vi "BangBang_GetAll.vi"(11 "BANG_BANG":T1 {"Measurment" format="%13.5p"; "Setpoint" format="%13.5p"; "Tolerance" format="%13.5p"}) -> (1 "Tolerance":dbl, 2 "Measurment":dbl, 3 "Setpoint":dbl)   [LabVIEW 2019, in "Trajectory_Library.lvlib"]
doc: "Gets elements of the internal data cluster\n\nInput:\n - BangBang -- Data cluster\n\nOutput\n - Setpoint -- Current stored setpoint (SP)\n - Measurement -- Current stored process variable (PV)\n - Tolerance -- Current stored tolerance."
uses:
  Trajectory_Library.lvlib
  TypeDef/BANG_BANG.ctl
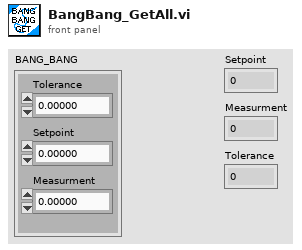
[diagram p1: front panel]
types:
  T1 = typedef "Trajectory_Library.lvlib/BANG_BANG.ctl" = cluster{"Tolerance":dbl, "Setpoint":dbl, "Measurment":dbl}
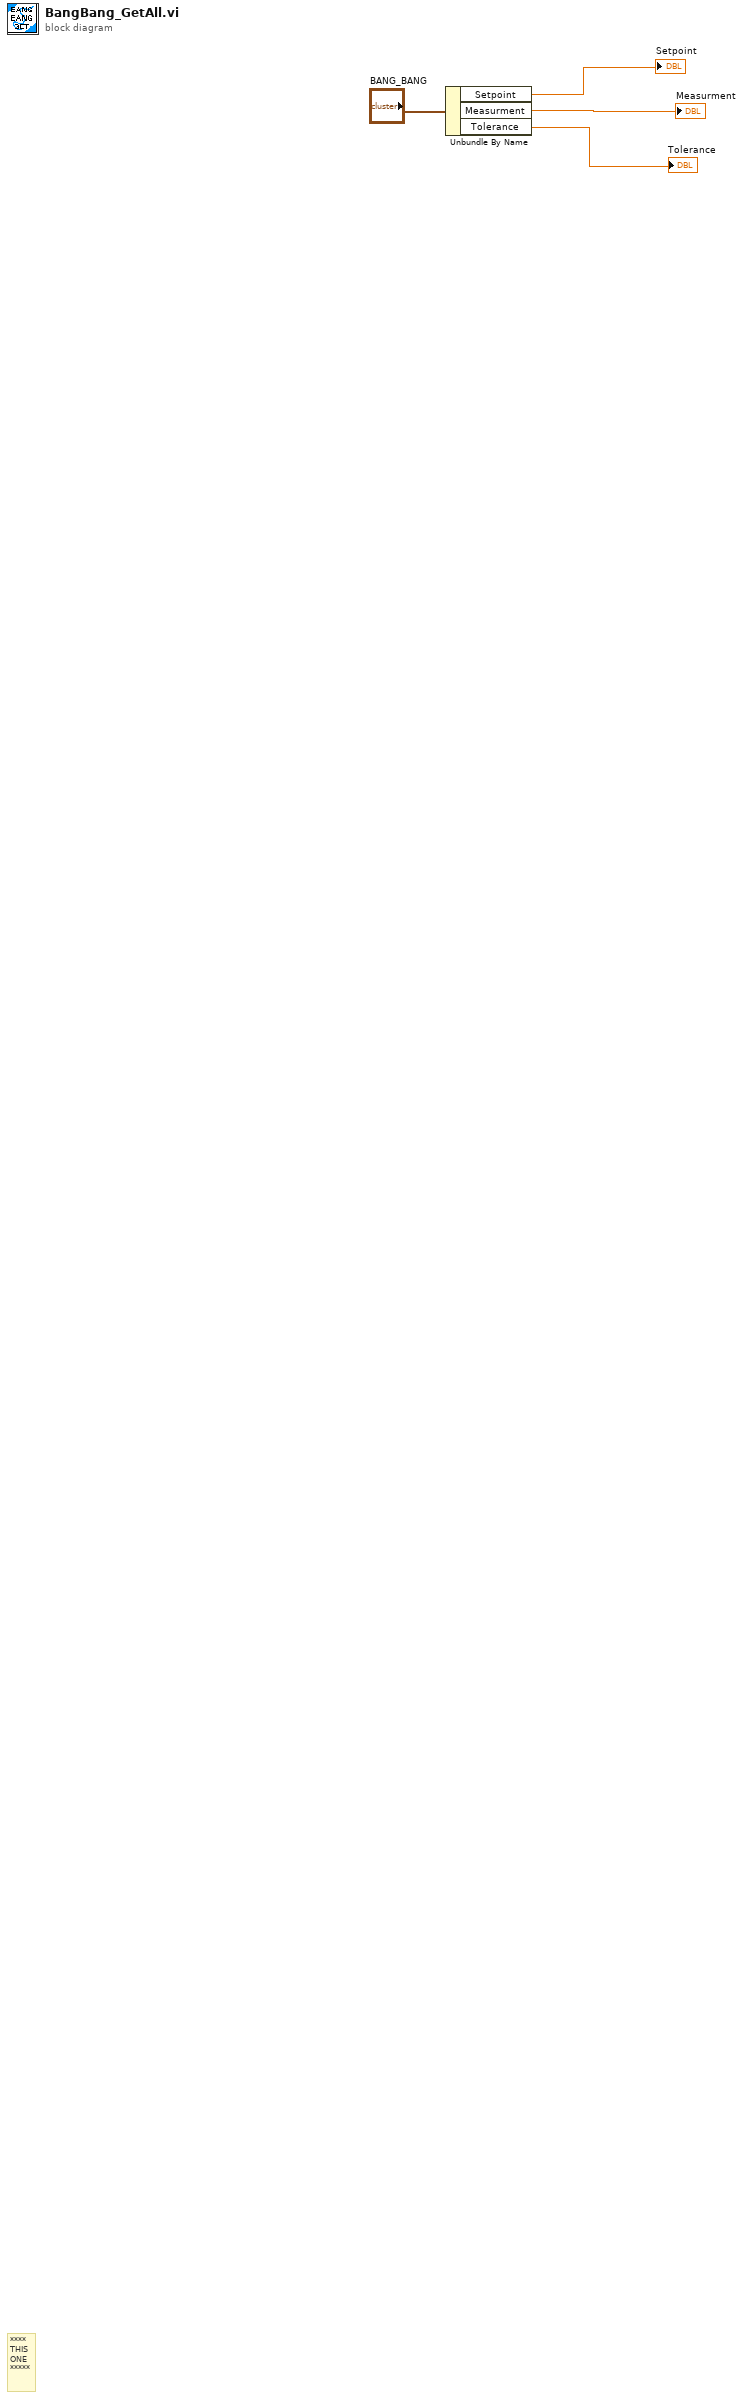
[diagram p0: block diagram]
diagram:
  # "****\nTHIS\nONE\n*****"
  n1 = Unbundle By Name("BANG_BANG") -> ("Setpoint"=→"Setpoint":dbl, "Measurment"=→"Measurment":dbl, "Tolerance"=→"Tolerance":dbl)
